vi "Session Console Entry.vi"(0 "Session Data In":T2={"MIDI-Messages"=[], "Rx-Data"=[], "Tx-Data"=[], "Session States"=enum."Wait to begin", "Tx Index"=0, "Communication Settings"={"Tx Protocol"=enum."Not Active", "Rx Protocol"=enum."Serial", "Serial"={"Tx Port"="", "Rx Port"="", "Baud rate"=8, "Parity"=enum."Space", "Data bits"=0, "Stop bits"=0, "Flow control"=enum."None", "Tx Resource"="", "Rx Resource"=""}, "MIDI Device"={"Input uDevice ID"=0, "Output uDevice ID"=0, "hmidiout Handle"=0, "hmidiin Handle"=0}, "Bluetooth"={"Dummy"=""}, "USB"={"Dummy"=""}}, "Timout-Time[ms]"=0, "Payload"=variant, "Queue_Session"=refnum, "To_GUI-Session"=refnum, "No More\nData"=FALSE, "Queue_Consumer"=refnum, "MIDI-Messages Log"=[], "Console log"=""}, 11 "Console Entry":string, 13 "Error In":errorcluster) -> (4 "Session Data 2":T2={"MIDI-Messages"=[], "Rx-Data"=[], "Tx-Data"=[], "Session States"=enum."Wait to begin", "Tx Index"=0, "Communication Settings"={"Tx Protocol"=enum."Not Active", "Rx Protocol"=enum."Serial", "Serial"={"Tx Port"="", "Rx Port"="", "Baud rate"=8, "Parity"=enum."Space", "Data bits"=0, "Stop bits"=0, "Flow control"=enum."None", "Tx Resource"="", "Rx Resource"=""}, "MIDI Device"={"Input uDevice ID"=0, "Output uDevice ID"=0, "hmidiout Handle"=0, "hmidiin Handle"=0}, "Bluetooth"={"Dummy"=""}, "USB"={"Dummy"=""}}, "Timout-Time[ms]"=0, "Payload"=variant, "Queue_Session"=refnum, "To_GUI-Session"=refnum, "No More\nData"=FALSE, "Queue_Consumer"=refnum, "MIDI-Messages Log"=[], "Console log"=""})   [LabVIEW 2019]
doc: "Adds a new entry to a console log, if an error has occured it will also be logged."
uses:
  Controls/Session_Data.ctl
  MIDI/Controls/MIDI-Message_Array.ctl
  MIDI/Controls/MIDI-Message_Cluster.ctl
  MIDI/Controls/Meta_Commands.ctl
  Controls/Session_State.ctl
  Common/Controls/Communication_Settings.ctl
  Common/Controls/Communication_Protocols.ctl
  Common/Controls/Application_Message.ctl
  Common/Controls/Application_State.ctl
panel:
  in  "Tab Control":T1(tab)
  out "Console log in":string
  out "Timestamp":string
  out "Console log out":string
  out "VI-filename":string
  out "VI Path":path
  out "Code Size":u32
  out "Revision Number":u32
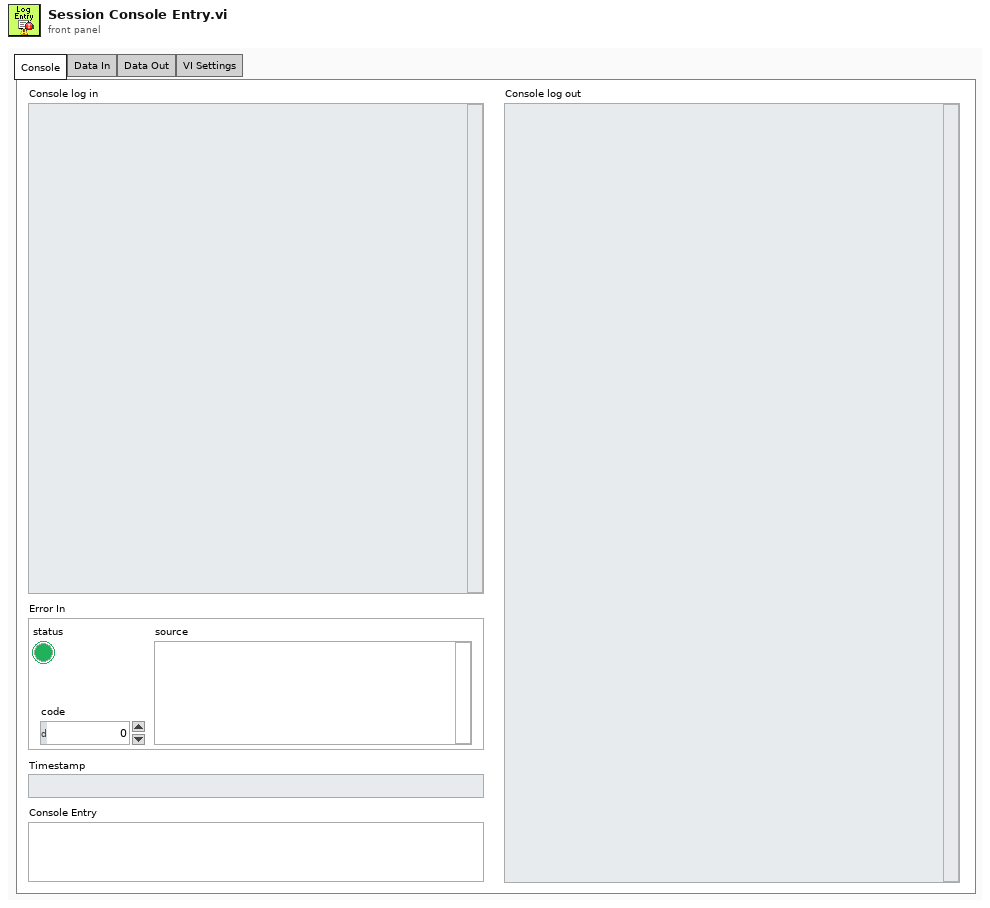
[diagram p1: front panel]
types:
  T1 = enum32{"Console", "Data In", "Data Out", "VI Settings"}
  T2 = typedef "Session_Data.ctl" = cluster{"MIDI-Messages":T3, "Rx-Data":i8[], "Tx-Data":i8[], "Session States":T6, "Tx Index":i32, "Communication Settings":T7, "Timout-Time[ms]":i32, "Payload":variant, "Queue_Session":refnum<queue>, "To_GUI-Session":refnum<user-event>, "No More\nData":bool, "Queue_Consumer":refnum<queue>, "MIDI-Messages Log":T3, "Console log":string}
  T3 = typedef "MIDI-Message_Array.ctl" = T4[]
  T4 = typedef "MIDI-Message_Cluster.ctl" = cluster{"Message Name":string, "Meta value":i32, "Datastring":string, "Datatype":T5}
  T5 = typedef "Meta_Commands.ctl" = enum16{"No Data", "Pause", "Loop", "Wait for Rx", "Delay", "Break", "MIDI"}
  T6 = typedef "Session_State.ctl" = enum16{"Wait to begin", "Active Session", "Pause", "Wait for Response", "Stop", "Restart", "Inspect", "Exit"}
  T7 = typedef "Communication_Settings.ctl" = cluster{"Tx Protocol":T8, "Rx Protocol":T8, "Serial":cluster{"Tx Port":refnum<visa-resource-name>, "Rx Port":refnum<visa-resource-name>, "Baud rate":i32, "Parity":enum16{"None", "Odd", "Even", "Mark", "Space"}, "Data bits":i32, "Stop bits":i32, "Flow control":enum16{"None", "XON/XOFF", "RTS/CTS", "XON/XOFF & RTS/CTS", "DTR/DSR", "XON/XOFF & DTR/DSR"}, "Tx Resource":refnum<visa-resource-name>, "Rx Resource":refnum<visa-resource-name>}, "MIDI Device":cluster{"Input uDevice ID":u32, "Output uDevice ID":u32, "hmidiout Handle":i32, "hmidiin Handle":i32}, "Bluetooth":cluster{"Dummy":string}, "USB":cluster{"Dummy":string}}
  T8 = typedef "Communication_Protocols.ctl" = enum16{"Serial", "Bluetooth", "USB-MIDI", "MIDI (Audio Device)", "Not Active"}
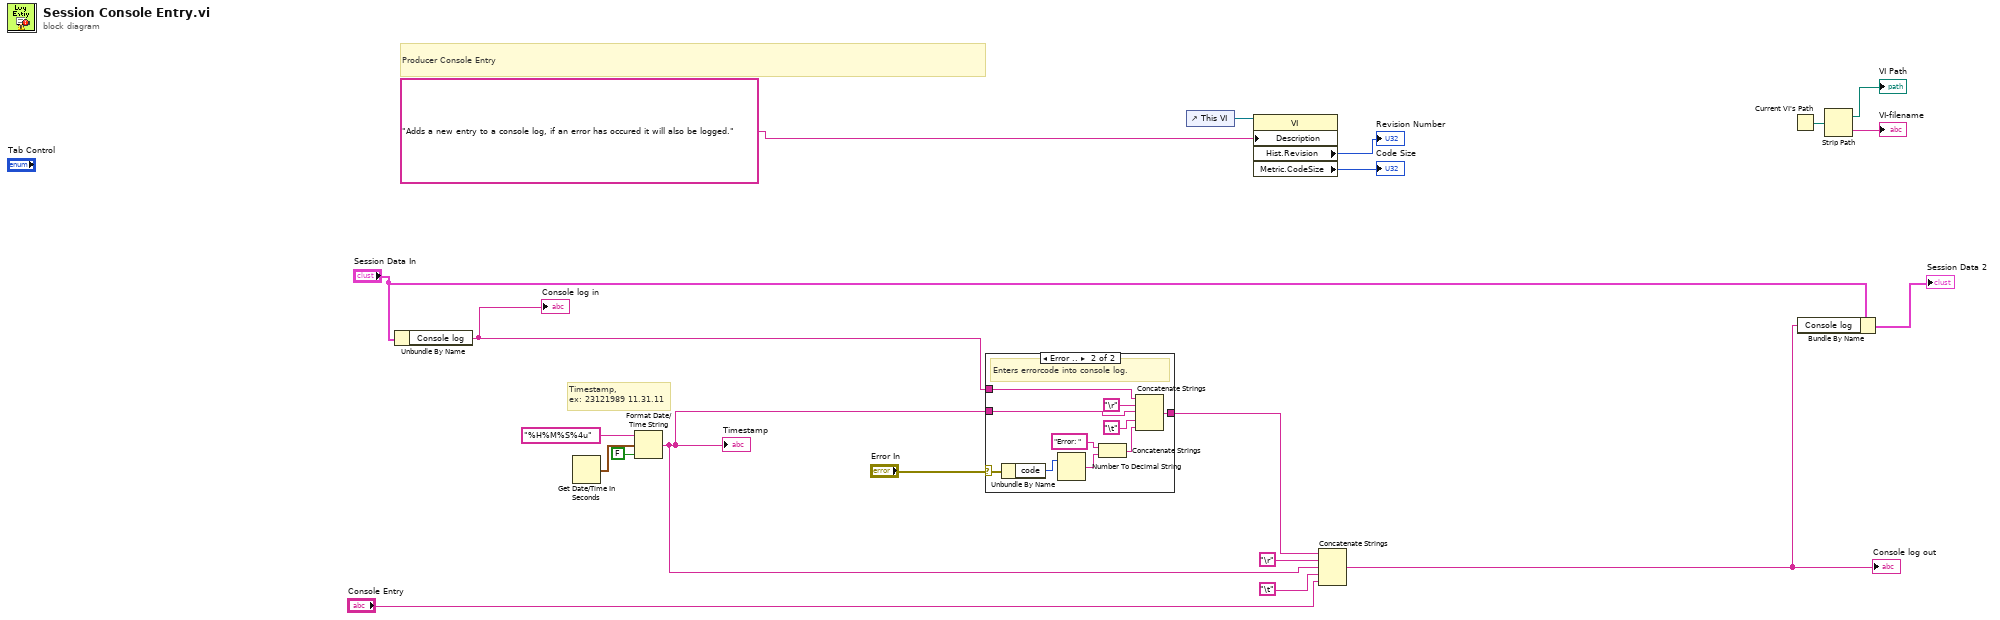
[diagram p0: block diagram]
diagram:
  # "Timestamp, \nex: 23121989 11.31.11"
  # "Producer Console Entry"
  n1 = Unbundle By Name("Session Data In") -> ("Console log"=w9:string)
  "Console log in" <- w9
  n2 = Get Date/Time In Seconds() -> (seconds since 1Jan1904=w13:timestamp)
  n3 = Format Date/Time String(time format string (%c)="%H%M%S%4u", seconds (now)=w13, UTC format=FALSE) -> (date/time string=w8:string)
  "Timestamp" <- w8
  n4 = case shown="Error .." "Error In" {
    selector: "Error In" -> [_ w22]
    tunnel: w9 -> [w21 w27]
    tunnel: w8 -> [_ w25]
    tunnel: [w21 w23] -> w7
    frame No Error {
    }
    frame Error {
      # "Enters errorcode into console log."
      n5 = Unbundle By Name(w22) -> ("code"=w31:i32)
      n6 = Number To Decimal String(number=w31) -> (decimal integer string=w30:string)  [unwired: 1 in]
      n7 = Concatenate Strings("Error: " ("string"), w30) -> (w29:string)
      n8 = Concatenate Strings(w27, "\r", w25, "\t", w29) -> (w23:string)
    }
  }
  n9 = control-ref of="This VI"() -> (w4:refnum<vi>)
  n10 = property class="VI"(reference=w4, "Description"="Adds a new entry to a console log, if an error has occured it will also be logged.") -> ("Hist.Revision"=→"Revision Number":u32, "Metric.CodeSize"=→"Code Size":u32)  [unwired: 1 in, 2 out]
  n11 = Concatenate Strings(w7, "\r", w8, "\t", "Console Entry") -> (w16:string)
  "Console log out" <- w16
  n12 = Current VI's Path() -> (path=w20:path)
  n13 = Bundle By Name(cluster="Session Data In", "Console log"=w16) -> (→"Session Data 2":T2)
  n14 = Strip Path(path=w20) -> (stripped path=→"VI Path":path, name=→"VI-filename":string)
